vi "IPI_LaserStringFormat.vi"(11 "响应":string) -> (0 "Value":dbl, 3 "连接的字符串":string)   [LabVIEW 2015]
panel:
  out "子字符串 3":string
  out "字符串 3":string
  out "4":bool
  out "3":bool
  out "数字":u32
  out "添加的数组":bool[](array[boolean])
  out "字符串 2":string
  out "数组 3":bool[](array[boolean])
  out "字符串":string
  out "数组 2":string[](array[string])
  out "数组":string[](array[string])
  out "子字符串 2":string
  out "子字符串":string
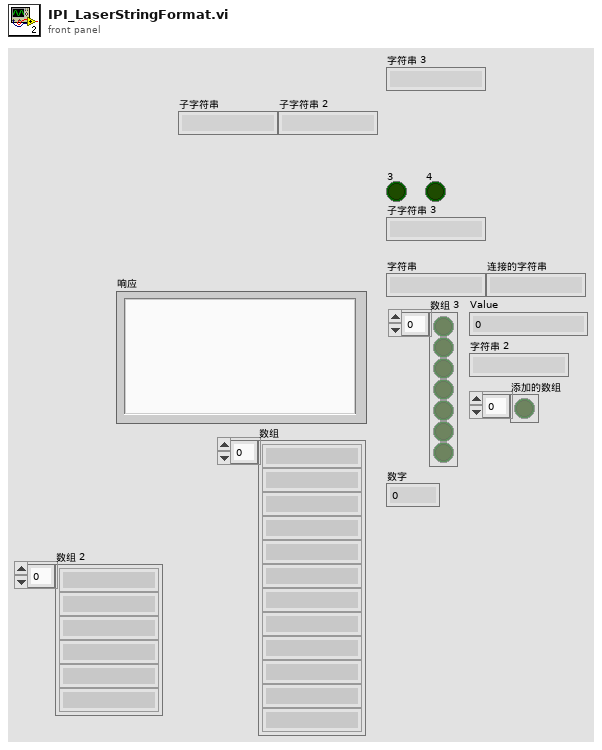
[diagram p1: front panel]
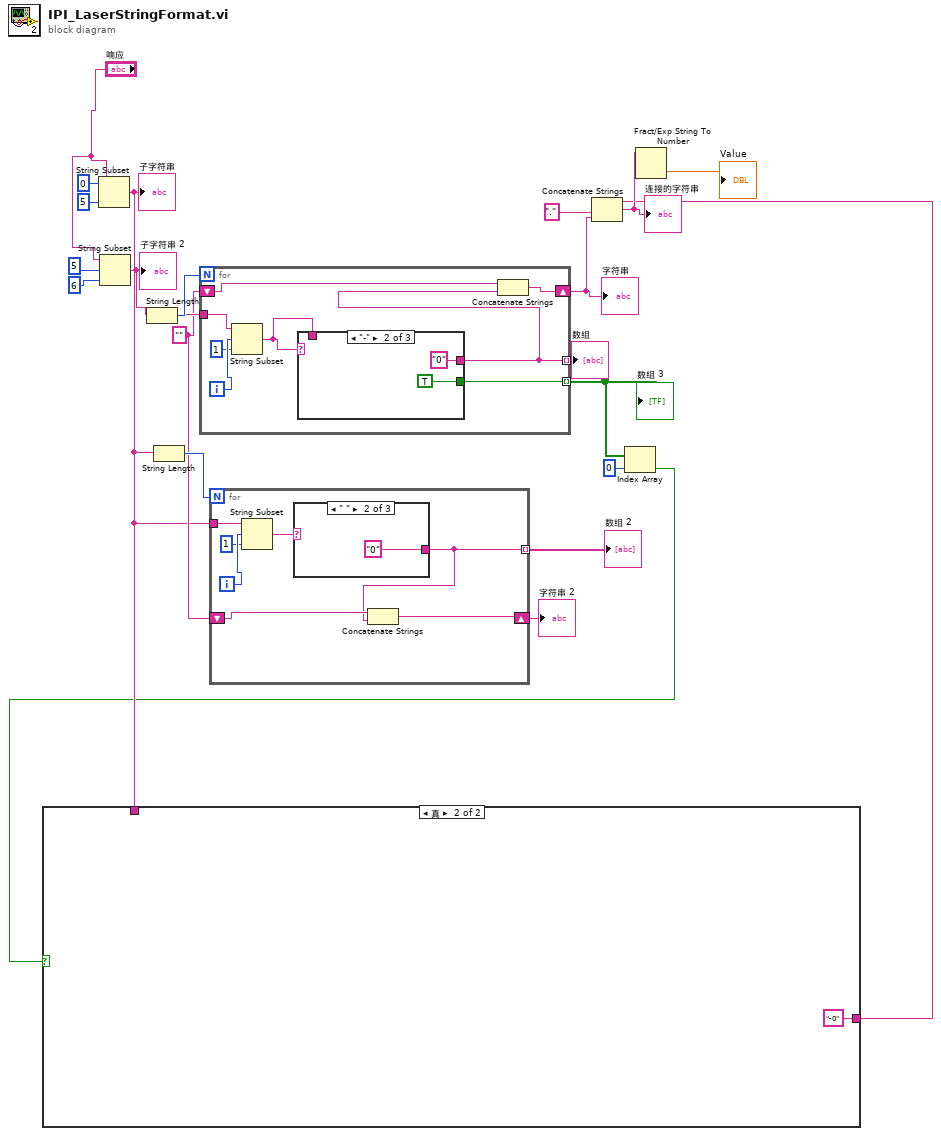
[diagram p0: block diagram]
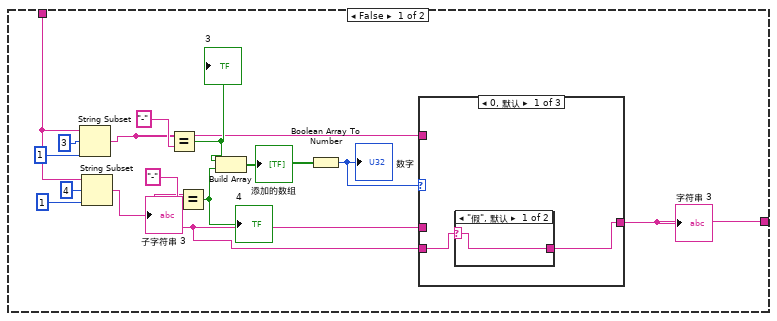
[diagram p2: hidden frame]
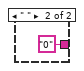
[diagram p3: hidden frame]
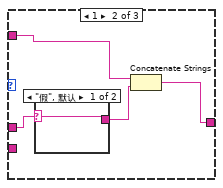
[diagram p4: hidden frame]
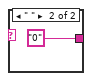
[diagram p5: hidden frame]
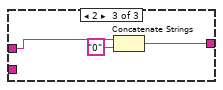
[diagram p6: hidden frame]
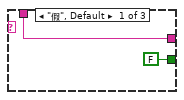
[diagram p9: hidden frame]
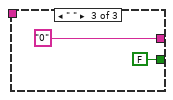
[diagram p10: hidden frame]
diagram:
  w7 = ""
  n1 = String Subset(string="响应", offset (0)=0 ("偏移量(0)"), length (rest)=5 ("长度（剩余）")) -> (substring=w5:string)
  "子字符串" <- w5
  n2 = String Subset(string="响应", offset (0)=5 ("偏移量(0)"), length (rest)=6 ("长度（剩余）")) -> (substring=w14:string)
  "子字符串 2" <- w14
  n3 = String Length(string=w14) -> (length=w16:i32)
  n4 = String Length(string=w5) -> (length=w13:i32)
  n5 = for {
    N: w16 -> [_]
    tunnel: [w25] -> w15 mode=indexing
    tunnel: w14 -> [w27]
    shift-right: [w24] -> w10
    shift-left: w7 -> [w26]
    tunnel: [w22] -> w3 mode=indexing
    i -> [w29]
    n6 = String Subset(string=w27, offset (0)=w29, length (rest)=1 ("长度（剩余）")) -> (substring=w23:string)
    n7 = case shown="\"-\"" w23 {
      tunnel: [w31 "0" ("y") "0" ("y")] -> w25
      tunnel: w23 -> [w31 _ _]
      tunnel: [FALSE TRUE FALSE] -> w22
      frame "假", Default {
      }
      frame "-" {
      }
      frame " " {
      }
    }
    n8 = Concatenate Strings(w26, w25) -> (w24:string)
  }
  "数组" <- w15
  "字符串" <- w10
  "数组 3" <- w3
  n9 = for {
    N: w13 -> [_]
    tunnel: w5 -> [w40]
    tunnel: [w37] -> w12 mode=indexing
    shift-right: [w36] -> w6
    shift-left: w7 -> [w38]
    i -> [w42]
    n10 = String Subset(string=w40, offset (0)=w42, length (rest)=1 ("长度（剩余）")) -> (substring=w39:string)
    n11 = case shown="\" \"" w39 {
      selector: w39 -> [w43 _ w45]
      tunnel: [w43 "0" w45] -> w37
      frame "假", Default {
      }
      frame " " {
      }
      frame "-" {
      }
    }
    n12 = Concatenate Strings(w38, w37) -> (w36:string)
  }
  "数组 2" <- w12
  "字符串 2" <- w6
  n13 = Index Array(array=w3, index=0 ("索引")) -> (element=w1:bool)
  n14 = case shown="真" w1 {
    tunnel: w5 -> [w55 _]
    tunnel: [w47 "-0"] -> w4
    frame False {
      n15 = String Subset(string=w55, offset (0)=3 ("偏移量(0)"), length (rest)=1 ("长度（剩余）")) -> (substring=w48:string)
      n16 = String Subset(string=w55, offset (0)=4 ("偏移量(0)"), length (rest)=1 ("长度（剩余）")) -> (substring=w46:string)
      "子字符串 3" <- w46
      n17 = Equal?(x=w48, y="-") -> (x = y?=w52:bool)
      "3" <- w52
      n18 = Equal?(x=w46, y="-") -> (x = y?=w51:bool)
      "4" <- w51
      n19 = Build Array(w52, w51) -> (w50:bool[])
      "添加的数组" <- w50
      n20 = Boolean Array To Number(Boolean array=w50) -> (number=w49:u32)
      "数字" <- w49
      n21 = case shown="0, 默认" w49 {
        tunnel: w46 -> [_ w66 w72]
        tunnel: [w60 w64 w70] -> w47
        tunnel: w48 -> [_ w67 _]
        tunnel: w46 -> [w61 _ _]
        frame 0, Default {
          n22 = case shown="\"假\", 默认" w61 {
            selector: w61 -> [w62 _]
            tunnel: [w62 "0"] -> w60
            frame "假", Default {
            }
            frame " " {
            }
          }
        }
        frame 1 {
          n23 = case shown="\"假\", 默认" w66 {
            selector: w66 -> [w68 _]
            tunnel: [w68 "0"] -> w65
            frame "假", Default {
            }
            frame " " {
            }
          }
          n24 = Concatenate Strings(w67, w65) -> (w64:string)
        }
        frame 2 {
          n25 = Concatenate Strings(w72, "0" ("字符串")) -> (w70:string)
        }
      }
      "字符串 3" <- w47
    }
    frame True {
    }
  }
  n26 = Concatenate Strings(w4, ".", w10) -> (w9:string)
  "连接的字符串" <- w9
  n27 = Fract/Exp String To Number(string=w9) -> (number=→"Value":dbl)  [unwired: 3 in, 1 out]
